vi "Pose_Plus.vi"(9 "other TRANSFORM":T4, 11 "in POSE":T1) -> (3 "out POSE":T1)   [LabVIEW 2019, in "Trajectory_Library.lvlib"]
doc: "Transforms the pose by the given transformation and returns the new transformed pose. \"plus\" is the same as \"transformBy\"\n\nThe matrix multiplication is as follows\n [x_new] [cos, -sin, 0][transform.x]\n [y_new] += [sin, cos, 0][transform.y]\n [t_new] [0, 0, 1][transform.t]\n\nParameters:\n - IN POSE - The input POSE data structure\n - OTHER TRANSFORM - The transform to transform the pose by.\n\nReturn:\n - OUT POSE - The transformed pose."
uses:
  Trajectory_Library.lvlib
  POSE2D.ctl
  TRANSLATION2D.ctl
  ROTATION2D.ctl
  TRANSFORM2D.ctl
  Translation_RotateBy.vi
  Translation_Plus.vi
  Rotation_Plus.vi
  Pose_New_TRRO.vi
  Translation_Create.vi
  Rotation_RotateBy.vi
  Rotation_CreateXY.vi
  Util_CalcDist.vi
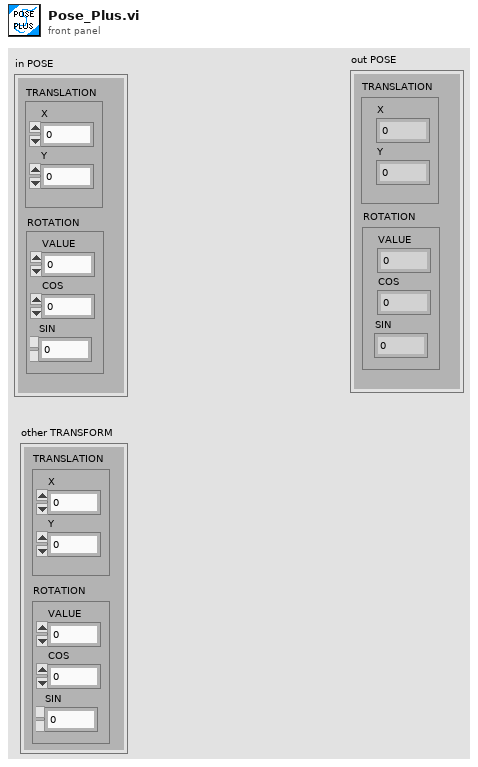
[diagram p1: front panel]
types:
  T1 = typedef "Trajectory_Library.lvlib/POSE2D.ctl" = cluster{"TRANSLATION":T2, "ROTATION":T3}
  T2 = typedef "Trajectory_Library.lvlib/TRANSLATION2D.ctl" = cluster{"X":dbl, "Y":dbl}
  T3 = typedef "Trajectory_Library.lvlib/ROTATION2D.ctl" = cluster{"VALUE":dbl, "COS":dbl, "SIN":dbl}
  T4 = typedef "Trajectory_Library.lvlib/TRANSFORM2D.ctl" = cluster{"TRANSLATION":T2, "ROTATION":T3}
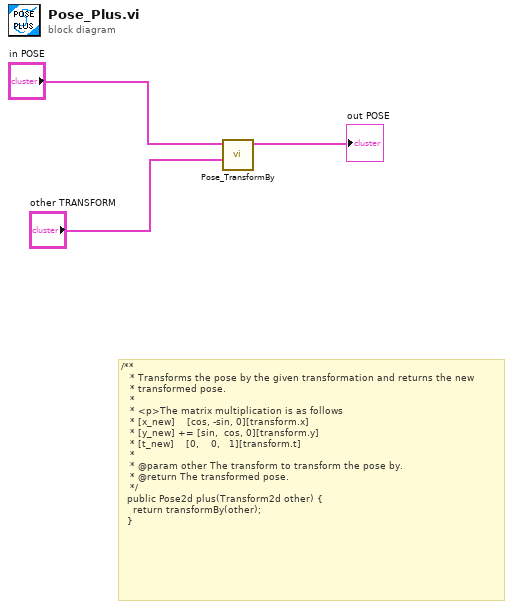
[diagram p0: block diagram]
diagram:
  # "/**\n   * Transforms the pose by the given transformation and returns the new\n   * transformed pose.\n   *\n   * <p>The matrix multiplication is as follows\n   * [x_new]    [cos, -sin, 0][transform.x]\n   * [y_new] += [sin,  cos, 0][transform.y]\n   * [t_new]    [0,    0,   1][transform.t]\n   *\n   * @param other The transform to transform the pose by.\n   * @return The transformed pose.\n   */\n  public Pose2d plus(Transform2d other) {\n    return transformBy(other);\n  }"
  n1 = call "Pose_TransformBy.vi"("other TRANSFORM"="other TRANSFORM", "in POSE"="in POSE") -> ("out POSE"=→"out POSE":T1)  [unwired: 9 in]
